vi "PH_PowerUnit_BaseClass.check Conditions.vi"(0 "VI in":refnum<vi>, 5 "error in (no error)":errorcluster) -> (14 "VI out":refnum<vi>, 17 "Ready for shot":bool, 18 "Ready to switch PU on":bool, 19 "error out":errorcluster)   [LabVIEW 2014, in "PH_PowerUnit_BaseClass.lvlib"]
uses:
  PH_PowerUnit_BaseClass.lvlib
  PH_SystemInformation/PH_SystemInformationEnabling State.ctl
  PH_StatusHandler/PH_StatusHandler.Status.ctl
  PH_SystemInformation/PH_SystemInformation.lvlib
  PH_StatusHandler/PH_StatusHandler.lvlib
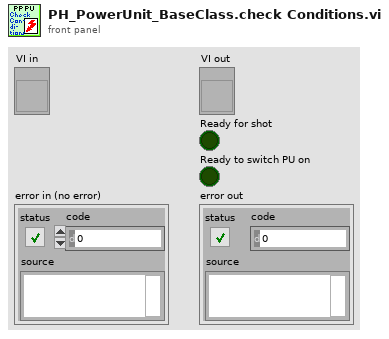
[diagram p1: front panel]
types:
  T1 = typedef "PH_StatusHandler.lvlib/PH_StatusHandler.Status.ctl" = i16
  T2 = typedef "PH_SystemInformation.lvlib/PH_SystemInformationEnabling State.ctl" = i32
  T3 = typedef "PH_PowerUnit_BaseClass.lvlib/PH_PowerUnit_BaseClass.i attribute.ctl" = cluster{"Constructor finished":bool, "PU":cluster{"In use":bool, "Service ID in use":i32, "GUI Ref":refnum<vi>}, "Enabling":cluster{"State":T2, "GUI Ref":refnum<vi>}, "Timing":cluster{"Last Shot":dbl, "Time between Shots [Sec]":dbl, "Waiting Time over?":bool, "Service ID Waiting Time":i32, "GUI Ref":refnum<vi>, "Instance":cluster{"Status":T1, "linked?":bool, "GUI Ref":refnum<vi>}}, "Sequencer":cluster{"SM State":string, "GUI Ref":refnum<vi>, "linked":bool}, "Subscribed Trendmssgs":cluster{"Tagname":string, "Status":T1, "linked?":bool, "Shot Condition":T1, "GUI Ref":refnum<vi>}[], "PP PU":T4, "Default Voltage (V)":dbl, "GUI Refs":T5, "PSDB data":cluster{"Shot Voltage [V]":dbl, "State TO SM":T6, "Write 2 early":bool}, "State TO SM":T6}
  T4 = typedef "PH_PP_Common.lvlib/PH_PP_Common.PUs.ctl" = enum16{"no Info", "PA-19mm-1", "PA-19mm-2", "PA-45mm-PILC", "PA-45mm-MAIN", "MA-PU-1", "MA-PU-2", "MA-PU-3", "MA-PU-4", "MA-PU-5", "MA-PU-6", "MA-FR", "MA-PILC", "PA-45mm-DP"}
  T5 = typedef "PH_PowerUnit_BaseClass.lvlib/PH_PowerUnit_BaseClass.GUI Refs.ctl" = cluster{"Delete Inst":refnum<vi>, "State TO SM":refnum<vi>, "State SM":refnum<vi>, "Fire":refnum<vi>}
  T6 = typedef "PH_PowerUnit_BaseClass.lvlib/PH_PowerUnit_BaseClass.SM States.ctl" = enum16{".", "Stand by", "Switch PU on", "Configure", "Set Default Voltage", "Set STANDBY", "Set READY", "Wait for Shot Cmd", "Open Dump Rods", "Open Ross Relais", "Close Ross Relais", "Switch PSU on", "Switch PSU off", "Charge", "Switch GD Channel on", "Close Dump Rods", "Rods-TO", "RR-TO", "PSU-TO", "Trigger-TO"}
  T7 = cluster{"Tagname":string, "Status":T1, "linked?":bool, "Shot Condition":T1, "GUI Ref":refnum<vi>}[]
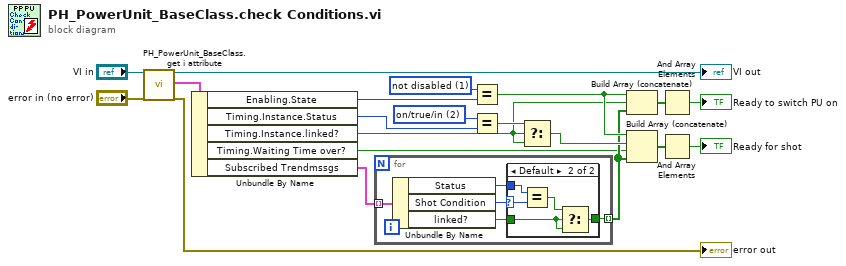
[diagram p0: block diagram]
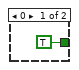
[diagram p2: hidden frame]
diagram:
  w8 = T1 2 items=["no info", "off/false/out", "on/true/in", "Failure", "Alarm", "Status 1", "Status 2", "Status 3"] ("y")
  w18 = T2 1 items=["no info", "not disabled", "disabled"] ("MainAmp Enabling State")
  n1 = call "PH_PowerUnit_BaseClass.get i attribute.vi"("i ref in"="VI in", "error in (no error)"="error in (no error)") -> ("i ref out"=→"VI out":refnum<vi>, "i attribute"=w15:T3, "error out"=→"error out":errorcluster)  [unwired: 15 in]
  n2 = Unbundle By Name(w15) -> ("Enabling.State"=w17:T2, "Timing.Instance.Status"=w9:T1, "Timing.Instance.linked?"=w4:bool, "Timing.Waiting Time over?"=w5:bool, "Subscribed Trendmssgs"=w1:T7)
  n3 = for {
    tunnel: w1 -> [w25] mode=indexing
    tunnel: [w21] -> w6 mode=indexing
    n4 = Unbundle By Name(w25) -> ("Status"=w23:T1, "Shot Condition"=w24:T1, "linked?"=w22:bool)
    n5 = case shown="Default" w24 {
      selector: w24 -> [_ w30]
      tunnel: w22 -> [_ w31]
      tunnel: w23 -> [_ w29]
      tunnel: [TRUE ("linked?") w27] -> w21
      frame 0 {
      }
      frame Default {
        n6 = Equal?(x=w29, y=w30) -> (x = y?=w28:bool)
        n7 = Select(t=w28, s=w31, f=w31) -> (s? t:f=w27:bool)
      }
    }
  }
  n8 = Equal?(x=w18, y=w17) -> (x = y?=w7:bool)
  n9 = Equal?(x=w8, y=w9) -> (x = y?=w10:bool)
  n10 = Select(t=w10, s=w4, f=w4) -> (s? t:f=w12:bool)
  n11 = Build Array (concatenate)(w7, w4, w6) -> (w2:bool[])
  n12 = Build Array (concatenate)(w7, w12, w5, w6) -> (w19:bool[])
  n13 = And Array Elements(Boolean array=w2) -> (logical AND=→"Ready to switch PU on":bool)
  n14 = And Array Elements(Boolean array=w19) -> (logical AND=→"Ready for shot":bool)
